vi "Find Safe Path.vi"(7 "error in":errorcluster, 8 "Pos End":string, 9 "Pos Start":string, 10 "Config Folder":path) -> (0 "error out":errorcluster, 2 "Points Array":refnum<class "Vec3d Class.lvclass">[](array[class]))   [LabVIEW 2011]
uses:
  Vec3d Class/Vec3d Class.lvclass
  gVision API/gVision/gVision.lvlib
panel:
  in  "Num Points":i32
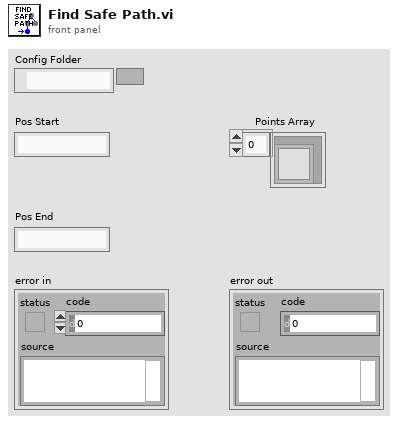
[diagram p1: front panel]
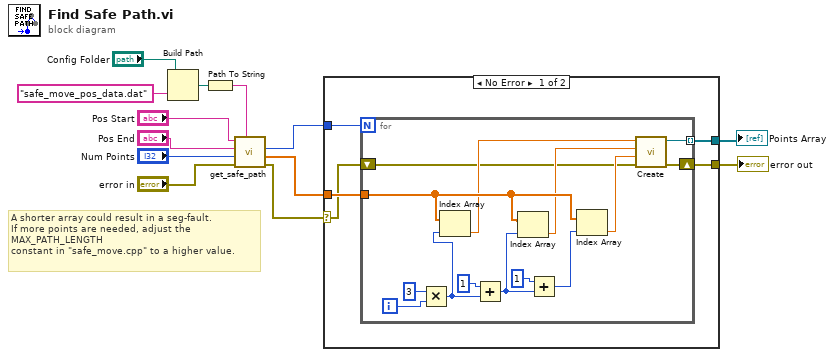
[diagram p0: block diagram]
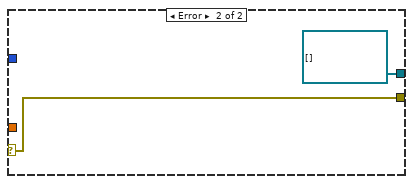
[diagram p2: hidden frame]
diagram:
  # "A shorter array could result in a seg-fault.\nIf more points are needed, adjust the\nMAX_PATH_LENGTH\nconstant in \"safe_move.cpp\" to a higher value."
  n1 = Build Path(base path="Config Folder", name or relative path="safe_move_pos_data.dat") -> (appended path=w9:path)
  n2 = Path To String(path=w9) -> (string=w5:string)
  n3 = call "get_safe_path.vi"("filename"=w5, "error in"="error in", "num_points"="Num Points", "end_label"="Pos End", "start_label"="Pos Start") -> ("error out"=w1:errorcluster, "coordinate_list"=w6:sgl[], "num_points out"=w7:i32)  [unwired: 4 in]
  n4 = case shown="No Error" w1 {
    selector: w1 -> [w14 w34]
    tunnel: [w18 refnum<class "Vec3d Class.lvclass">[] []] -> w13
    tunnel: [w17 w34] -> w12
    tunnel: w7 -> [w16 _]
    tunnel: w6 -> [w15 _]
    frame No Error {
      n5 = for {
        N: w16 -> [_]
        tunnel: w15 -> [w28]
        shift-right: [w19] -> w17
        shift-left: w14 -> [w20]
        tunnel: [w24] -> w18 mode=indexing
        i -> [w32]
        n6 = Multiply(x=3, y=w32) -> (x*y=w30:i32)
        n7 = Index Array(array=w28, index=w30) -> (element=w23:sgl)
        n8 = Add(x=1, y=w30) -> (x+y=w26:i32)
        n9 = Index Array(array=w28, index=w26) -> (element=w22:sgl)
        n10 = Add(x=1, y=w26) -> (x+y=w25:i32)
        n11 = Index Array(array=w28, index=w25) -> (element=w21:sgl)
        n12 = call "Create.vi"("error in"=w20, "Z"=w21, "Y"=w22, "X"=w23) -> ("error out"=w19:errorcluster, "Vec3d Class out"=w24:refnum<class "Vec3d Class.lvclass">)  [unwired: 6 in]
      }
    }
    frame Error {
    }
  }
  "error out" <- w12
  "Points Array" <- w13
